vi "BlkHeadRead.vi"(11 "引用句柄":refnum<file>) -> (0 "FramesPerStim":i32, 1 "datatype":i32, 2 "FrameHeight":i32, 3 "FrameWidth":i32, 4 "Stimuli":i32, 5 "SequenceOfID":u8[](array[numeric]))   [LabVIEW 2011]
panel:
  in  "错误输入":errorcluster
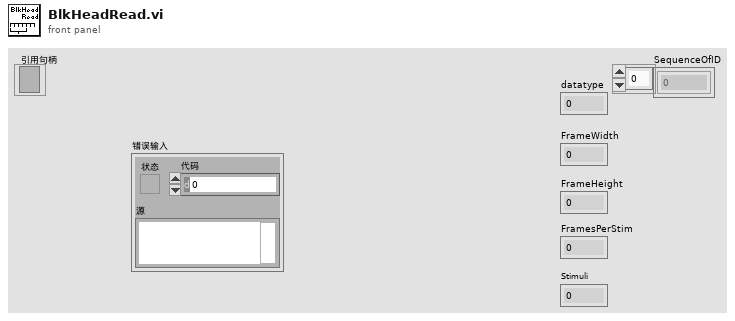
[diagram p1: front panel]
types:
  T1 = enum16{"big-endian, network order", "native, host order", "little-endian"}
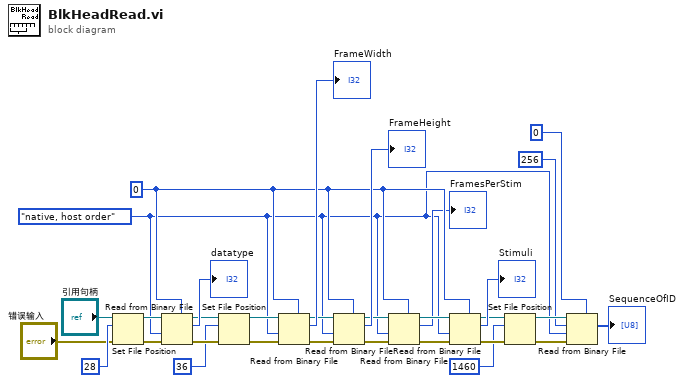
[diagram p0: block diagram]
diagram:
  w22 = 0 ("数值")
  w6 = T1."native, host order" ("字节顺序(0:big-endian, network order)")
  n1 = Set File Position(offset (in bytes) (0)=i64 28 ("偏移量（字节）（0）"), refnum="引用句柄", error in="错误输入") -> (refnum out=w12:refnum<file>, error out=w13:errorcluster)  [unwired: 1 in]
  n2 = Read from Binary File(5:w22, 8:w13, 9:w6, 11:w12) -> (0:w27:errorcluster, 2:→"datatype":i32, 3:w16:refnum<file>)  [unwired: 2 in, 1 out]
  n3 = Set File Position(offset (in bytes) (0)=i64 36 ("偏移量（字节）（0） 2"), refnum=w16, error in=w27) -> (refnum out=w17:refnum<file>, error out=w28:errorcluster)  [unwired: 1 in]
  n4 = Read from Binary File(5:w22, 8:w28, 9:w6, 11:w17) -> (0:w24:errorcluster, 2:→"FrameWidth":i32, 3:w14:refnum<file>)  [unwired: 2 in, 1 out]
  n5 = Read from Binary File(5:w22, 8:w24, 9:w6, 11:w14) -> (0:w25:errorcluster, 2:→"FrameHeight":i32, 3:w19:refnum<file>)  [unwired: 2 in, 1 out]
  n6 = Read from Binary File(5:w22, 8:w25, 9:w6, 11:w19) -> (0:w26:errorcluster, 2:→"FramesPerStim":i32, 3:w21:refnum<file>)  [unwired: 2 in, 1 out]
  n7 = Read from Binary File(5:w22, 8:w26, 9:w6, 11:w21) -> (0:w10:errorcluster, 2:→"Stimuli":i32, 3:w11:refnum<file>)  [unwired: 2 in, 1 out]
  n8 = Set File Position(offset (in bytes) (0)=i64 1460 ("偏移量（字节）（0）"), refnum=w11, error in=w10) -> (refnum out=w8:refnum<file>, error out=w7:errorcluster)  [unwired: 1 in]
  n9 = Read from Binary File(5:u8 0, 8:w7, 9:w6, 10:256 ("总数(1)"), 11:w8) -> (2:→"SequenceOfID":u8[])  [unwired: 1 in, 3 out]
